vi "PicoLogStart.vi"(1 "sampleInterval_ms":i32=1000, 2 "conversionTime":i16(ring) items=["60 ms", "100 ms", "180 ms", "340 ms", "660 ms"], 3 "Mains Frequency":i16(ring) items=["50 Hz", "60 Hz"], 9 "4":bool, 11 "5":bool) -> (12 "noOfChannels":i16=2, 13 "STOP":bool, 14 "handle":i16)   [LabVIEW 2014]
uses:
  Instance           1 22Saved   HRDL_streaming .vi
  Instance         138 22Saved   HRDL_streaming .vi
  picohrdl.dll
panel:
  in  "Ch nr":bool[](array[boolean])
  out "Unit Info":T1
  in  "13":bool
  in  "12":bool
  in  "11":bool
  in  "10":bool
  in  "9":bool
  in  "8":bool
  in  "7":bool
  in  "6":bool
  # "1       2       3      4       5        6       7       8       9      10     11      12     13    14       15     16"
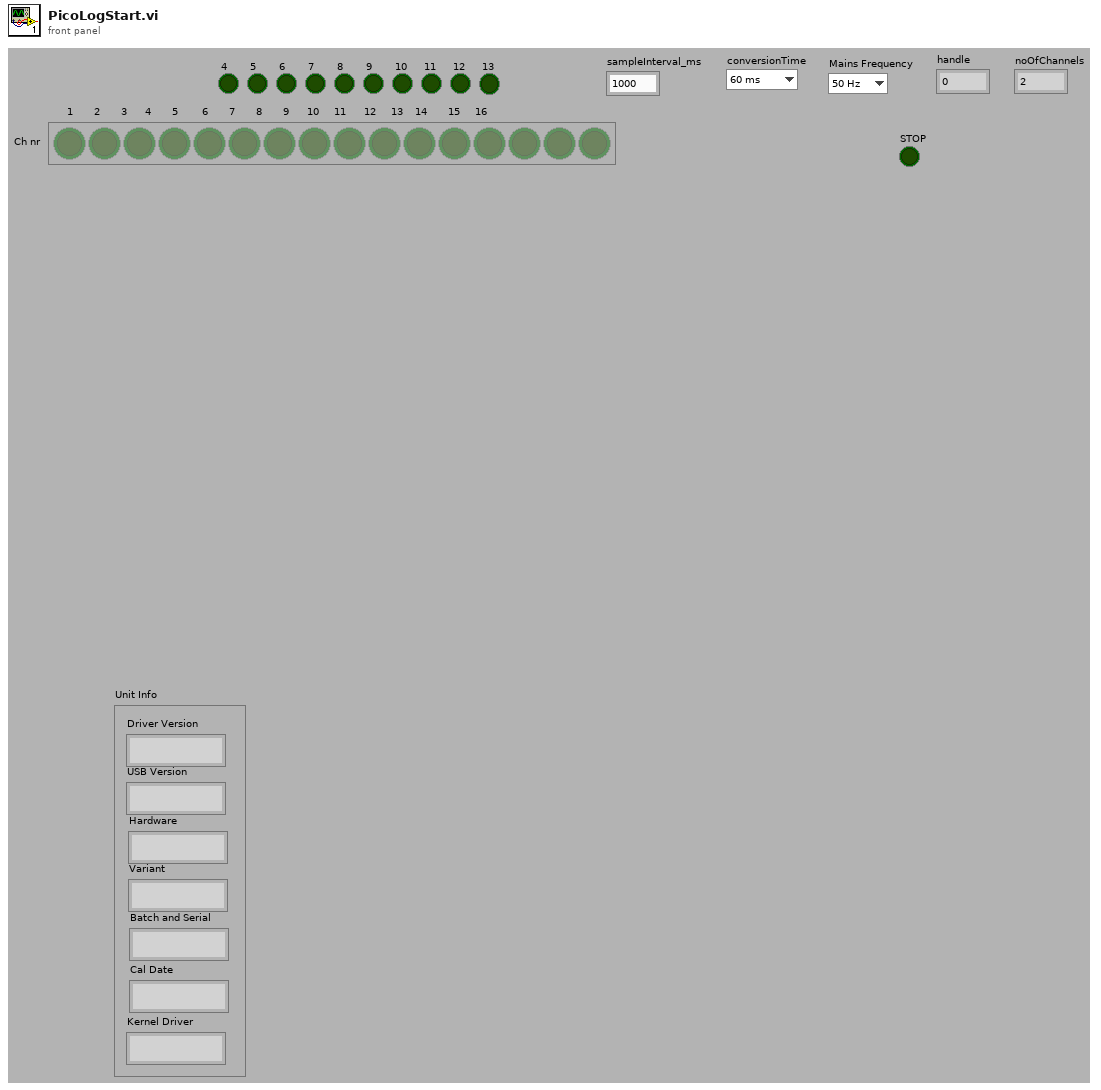
[diagram p1: front panel]
types:
  T1 = cluster{"Driver Version":string, "USB Version":string, "Hardware":string, "Variant":string, "Batch and Serial":string, "Cal Date":string, "Kernel Driver":string}
  T2 = cluster{"[0]":string, "[1]":string, "[2]":string, "[3]":string, "[4]":string, "[5]":string, "[6]":string}
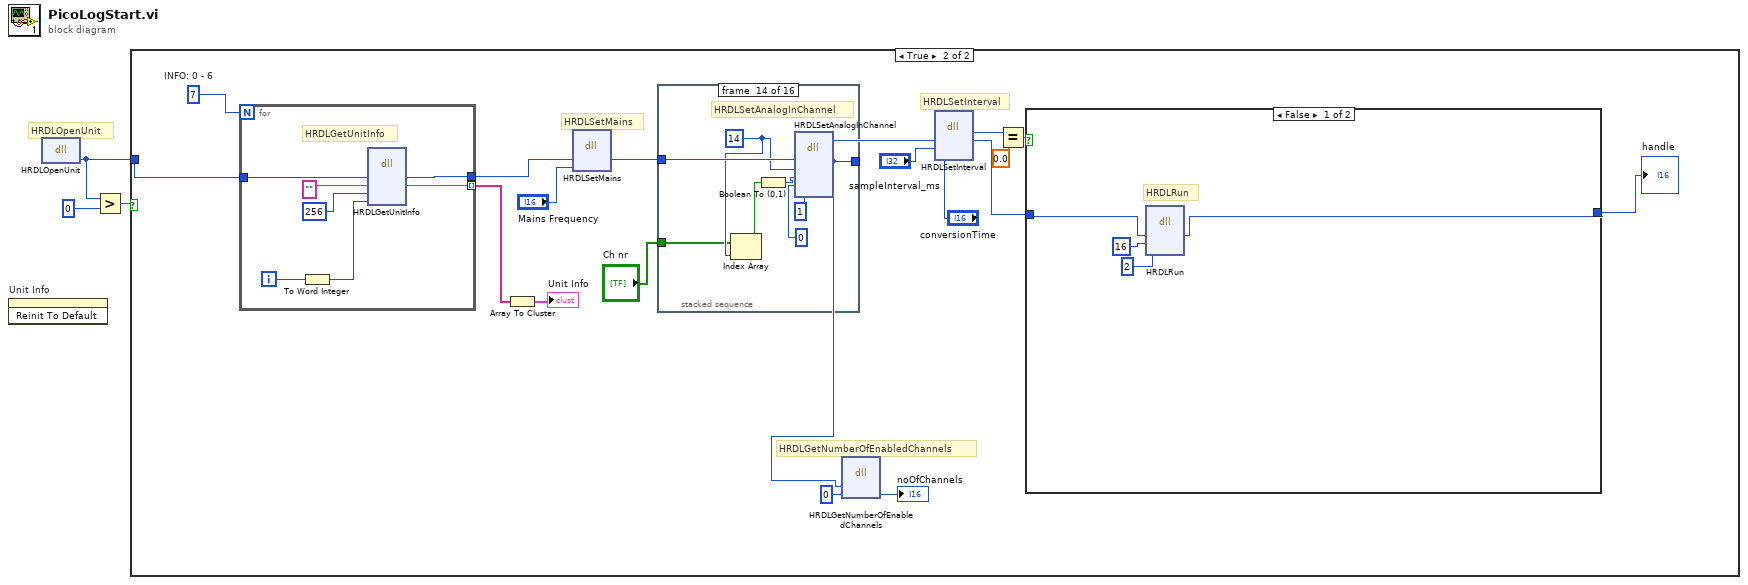
[diagram p0: block diagram]
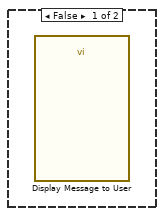
[diagram p2: hidden frame]
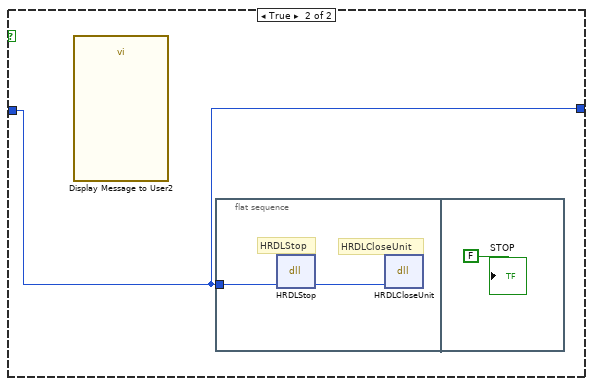
[diagram p3: hidden frame]
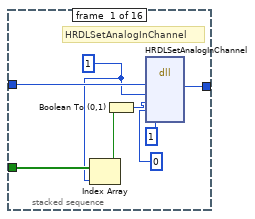
[diagram p4: hidden frame]
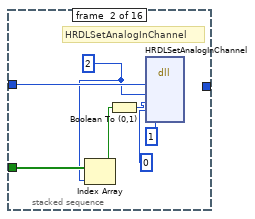
[diagram p5: hidden frame]
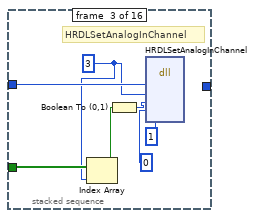
[diagram p6: hidden frame]
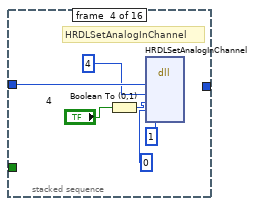
[diagram p7: hidden frame]
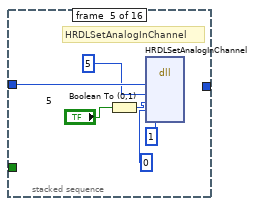
[diagram p8: hidden frame]
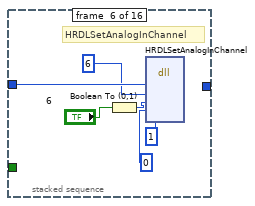
[diagram p9: hidden frame]
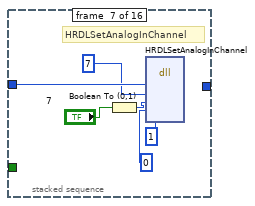
[diagram p10: hidden frame]
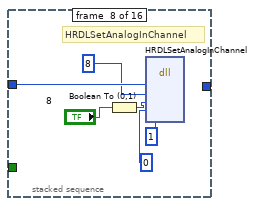
[diagram p11: hidden frame]
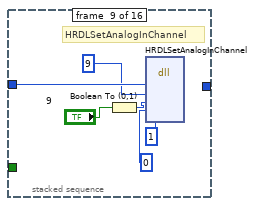
[diagram p12: hidden frame]
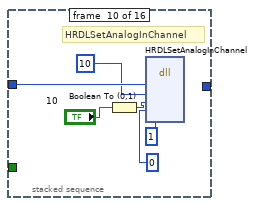
[diagram p13: hidden frame]
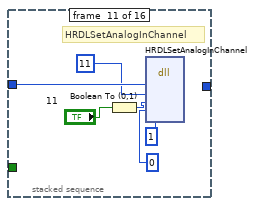
[diagram p14: hidden frame]
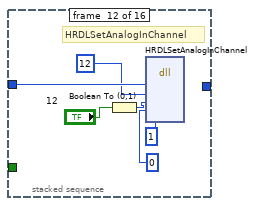
[diagram p15: hidden frame]
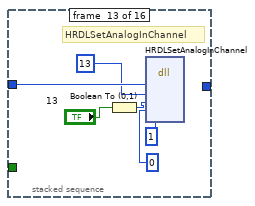
[diagram p16: hidden frame]
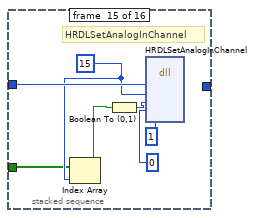
[diagram p17: hidden frame]
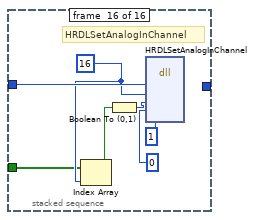
[diagram p18: hidden frame]
diagram:
  # "HRDLOpenUnit"
  n1 = invoke on="Unit Info" class="Clust (strict)" method="Reinit To Default"() -> ()  [unwired: 3 in, 3 out]
  n2 = dll-call lib="picohrdl.dll" fn="HRDLOpenUnit"() -> ("handle"=w1:i16)  [unwired: 3 in, 2 out]
  n3 = Greater?(x=w1, y=i16 0) -> (0:w3:bool)
  n4 = case shown="True" w3 {
    tunnel: w1 -> [_ w10]
    frame False {
      n5 = call "Display Message to User"() -> ()  [unwired: 10 in, 2 out]
    }
    frame True {
      w12 = 7  # INFO: 0 - 6
      # "HRDLGetNumberOfEnabledChannels"
      # "HRDLSetInterval"
      # "HRDLSetMains"
      n6 = for {
        N: w12 -> [_]
        tunnel: w10 -> [w28]
        tunnel: [w25] -> w9 mode=indexing
        tunnel: [w23] -> w11
        i -> [w24]
        # "HRDLGetUnitInfo"
        n7 = To Word Integer(number=w24) -> (16bit integer=w22:i16)
        n8 = dll-call lib="picohrdl.dll" fn="HRDLGetUnitInfo"("handle"=w28, "unitInfo"="", "stringLength"=i16 256, "info"=w22) -> ("handle"=w23:i16, "unitInfo"=w25:string)  [unwired: 6 in, 2 out]
      }
      n9 = Array To Cluster(array=w9) -> (cluster=→"Unit Info":T2)
      n10 = dll-call lib="PicoHRDL.dll" fn="HRDLSetMains"("handle"=w11, "sixtyHertz"="Mains Frequency") -> ("handle"=w14:i16)  [unwired: 5 in, 2 out]
      n11 = stacked-sequence {
        tunnel: w14 -> [w44 w51 w58 w64 w70 w76 w82 w88 w94 w100 w106 w112 w118 w125 w132 w139]
        tunnel: [w43 _ _ _ _ _ _ _ _ _ _ _ _ _ _ _] -> w13
        tunnel: "Ch nr" -> [w39 w47 w53 _ _ _ _ _ _ _ _ _ _ w119 w126 w133]
        frame #0 {
          w37 = i16 1 ("channel")
          # "HRDLSetAnalogInChannel"
          n12 = Index Array(array=w39, index=w37) -> (element=w38:bool)
          n13 = Boolean To (0,1)(Boolean=w38) -> (0, 1=w40:i16)
          n14 = dll-call lib="PicoHRDL.dll" fn="HRDLSetAnalogInChannel"("handle"=w44, "channel"=w37, "enabled"=w40, "range"=i16 0 ("range 1"), "singleEnded"=i16 1) -> ("handle"=w43:i16)  [unwired: 8 in, 2 out]
        }
        frame #1 {
          w45 = i16 2 ("channel")
          # "HRDLSetAnalogInChannel"
          n15 = Index Array(array=w47, index=w45) -> (element=w46:bool)
          n16 = Boolean To (0,1)(Boolean=w46) -> (0, 1=w48:i16)
          n17 = dll-call lib="PicoHRDL.dll" fn="HRDLSetAnalogInChannel"("handle"=w51, "channel"=w45, "enabled"=w48, "range"=i16 0 ("range 2"), "singleEnded"=i16 1) -> ()  [unwired: 9 in, 2 out]
        }
        frame #2 {
          w52 = i16 3 ("channel")
          # "HRDLSetAnalogInChannel"
          n18 = Index Array(array=w53, index=w52) -> (element=w54:bool)
          n19 = Boolean To (0,1)(Boolean=w54) -> (0, 1=w55:i16)
          n20 = dll-call lib="PicoHRDL.dll" fn="HRDLSetAnalogInChannel"("handle"=w58, "channel"=w52, "enabled"=w55, "range"=i16 0 ("range 3"), "singleEnded"=i16 1) -> ()  [unwired: 9 in, 2 out]
        }
        frame #3 {
          # "HRDLSetAnalogInChannel"
          n21 = Boolean To (0,1)(Boolean="4") -> (0, 1=w60:i16)
          n22 = dll-call lib="PicoHRDL.dll" fn="HRDLSetAnalogInChannel"("handle"=w64, "channel"=i16 4, "enabled"=w60, "range"=i16 0 ("range 4"), "singleEnded"=i16 1) -> ()  [unwired: 9 in, 2 out]
        }
        frame #4 {
          # "HRDLSetAnalogInChannel"
          n23 = Boolean To (0,1)(Boolean="5") -> (0, 1=w66:i16)
          n24 = dll-call lib="PicoHRDL.dll" fn="HRDLSetAnalogInChannel"("handle"=w70, "channel"=i16 5, "enabled"=w66, "range"=i16 0 ("range 5"), "singleEnded"=i16 1) -> ()  [unwired: 9 in, 2 out]
        }
        frame #5 {
          # "HRDLSetAnalogInChannel"
          n25 = Boolean To (0,1)(Boolean="6") -> (0, 1=w72:i16)
          n26 = dll-call lib="PicoHRDL.dll" fn="HRDLSetAnalogInChannel"("handle"=w76, "channel"=i16 6, "enabled"=w72, "range"=i16 0 ("range 6"), "singleEnded"=i16 1) -> ()  [unwired: 9 in, 2 out]
        }
        frame #6 {
          # "HRDLSetAnalogInChannel"
          n27 = Boolean To (0,1)(Boolean="7") -> (0, 1=w78:i16)
          n28 = dll-call lib="PicoHRDL.dll" fn="HRDLSetAnalogInChannel"("handle"=w82, "channel"=i16 7, "enabled"=w78, "range"=i16 0 ("range 7"), "singleEnded"=i16 1) -> ()  [unwired: 9 in, 2 out]
        }
        frame #7 {
          # "HRDLSetAnalogInChannel"
          n29 = Boolean To (0,1)(Boolean="8") -> (0, 1=w84:i16)
          n30 = dll-call lib="PicoHRDL.dll" fn="HRDLSetAnalogInChannel"("handle"=w88, "channel"=i16 8, "enabled"=w84, "range"=i16 0 ("range 8"), "singleEnded"=i16 1) -> ()  [unwired: 9 in, 2 out]
        }
        frame #8 {
          # "HRDLSetAnalogInChannel"
          n31 = Boolean To (0,1)(Boolean="9") -> (0, 1=w90:i16)
          n32 = dll-call lib="PicoHRDL.dll" fn="HRDLSetAnalogInChannel"("handle"=w94, "channel"=i16 9, "enabled"=w90, "range"=i16 0 ("range 9"), "singleEnded"=i16 1) -> ()  [unwired: 9 in, 2 out]
        }
        frame #9 {
          # "HRDLSetAnalogInChannel"
          n33 = Boolean To (0,1)(Boolean="10") -> (0, 1=w96:i16)
          n34 = dll-call lib="PicoHRDL.dll" fn="HRDLSetAnalogInChannel"("handle"=w100, "channel"=i16 10, "enabled"=w96, "range"=i16 0 ("range 10"), "singleEnded"=i16 1) -> ()  [unwired: 9 in, 2 out]
        }
        frame #10 {
          # "HRDLSetAnalogInChannel"
          n35 = Boolean To (0,1)(Boolean="11") -> (0, 1=w102:i16)
          n36 = dll-call lib="PicoHRDL.dll" fn="HRDLSetAnalogInChannel"("handle"=w106, "channel"=i16 11, "enabled"=w102, "range"=i16 0 ("range 11"), "singleEnded"=i16 1) -> ()  [unwired: 9 in, 2 out]
        }
        frame #11 {
          # "HRDLSetAnalogInChannel"
          n37 = Boolean To (0,1)(Boolean="12") -> (0, 1=w108:i16)
          n38 = dll-call lib="PicoHRDL.dll" fn="HRDLSetAnalogInChannel"("handle"=w112, "channel"=i16 12, "enabled"=w108, "range"=i16 0 ("range 12"), "singleEnded"=i16 1) -> ()  [unwired: 9 in, 2 out]
        }
        frame #12 {
          # "HRDLSetAnalogInChannel"
          n39 = Boolean To (0,1)(Boolean="13") -> (0, 1=w114:i16)
          n40 = dll-call lib="PicoHRDL.dll" fn="HRDLSetAnalogInChannel"("handle"=w118, "channel"=i16 13, "enabled"=w114, "range"=i16 0 ("range 13"), "singleEnded"=i16 1) -> ()  [unwired: 9 in, 2 out]
        }
        frame #13 {
          w120 = i16 14 ("channel")
          # "HRDLSetAnalogInChannel"
          n41 = Index Array(array=w119, index=w120) -> (element=w121:bool)
          n42 = Boolean To (0,1)(Boolean=w121) -> (0, 1=w122:i16)
          n43 = dll-call lib="PicoHRDL.dll" fn="HRDLSetAnalogInChannel"("handle"=w125, "channel"=w120, "enabled"=w122, "range"=i16 0 ("range 14"), "singleEnded"=i16 1) -> ()  [unwired: 9 in, 2 out]
        }
        frame #14 {
          w127 = i16 15 ("channel")
          # "HRDLSetAnalogInChannel"
          n44 = Index Array(array=w126, index=w127) -> (element=w128:bool)
          n45 = Boolean To (0,1)(Boolean=w128) -> (0, 1=w129:i16)
          n46 = dll-call lib="PicoHRDL.dll" fn="HRDLSetAnalogInChannel"("handle"=w132, "channel"=w127, "enabled"=w129, "range"=i16 0 ("range 15"), "singleEnded"=i16 1) -> ()  [unwired: 9 in, 2 out]
        }
        frame #15 {
          w134 = i16 16 ("channel")
          # "HRDLSetAnalogInChannel"
          n47 = Index Array(array=w133, index=w134) -> (element=w135:bool)
          n48 = Boolean To (0,1)(Boolean=w135) -> (0, 1=w136:i16)
          n49 = dll-call lib="PicoHRDL.dll" fn="HRDLSetAnalogInChannel"("handle"=w139, "channel"=w134, "enabled"=w136, "range"=i16 0 ("range 16"), "singleEnded"=i16 1) -> ()  [unwired: 9 in, 2 out]
        }
      }
      n50 = dll-call lib="PicoHRDL.dll" fn="HRDLGetNumberOfEnabledChannels"("handle"=w13, "nEnabledChannels"=i16 0) -> ("nEnabledChannels"=→"noOfChannels":i16)  [unwired: 5 in, 2 out]
      n51 = dll-call lib="PicoHRDL.dll" fn="HRDLSetInterval"("handle"=w13, "sampleInterval_ms"="sampleInterval_ms", "conversionTime"="conversionTime") -> ("return type"=w18:i16, "handle"=w17:i16)  [unwired: 5 in, 2 out]
      n52 = Equal?(x=w18, y=0.0) -> (x = y?=w16:bool)
      n53 = case shown="False" w16 {
        tunnel: [w29 w33] -> w7
        tunnel: w17 -> [w30 w33]
        frame False {
          # "HRDLRun"
          n54 = dll-call lib="PicoHRDL.dll" fn="HRDLRun"("handle"=w30, "nValues"=16, "method"=i16 2) -> ("handle"=w29:i16)  [unwired: 6 in, 2 out]
        }
        frame True {
          n55 = call "Display Message to User2"() -> ()  [unwired: 10 in, 2 out]
          n56 = flat-sequence {
            tunnel: w33 -> [w34]
            frame #0 {
              # "HRDLStop"
              # "HRDLCloseUnit"
              n57 = dll-call lib="picohrdl.dll" fn="HRDLStop"("handle"=w34) -> ("handle"=w35:i16)  [unwired: 4 in, 2 out]
              n58 = dll-call lib="PicoHRDL.dll" fn="HRDLCloseUnit"("handle"=w35) -> ()  [unwired: 5 in, 2 out]
            }
            frame #1 {
              "STOP" <- FALSE ("stop")
            }
          }
        }
      }
      "handle" <- w7
    }
  }
